vi "加速度_峰值.vi"(10 "信号X":dbl[](array[numeric]), 11 "n":i32) -> (3 "峰值":dbl)   [LabVIEW 2014]
uses:
  <vilib>/Analysis/NI_AAL_SigProc.lvlib
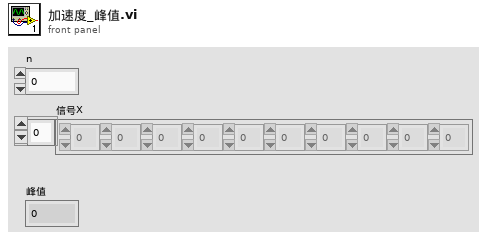
[diagram p1: front panel]
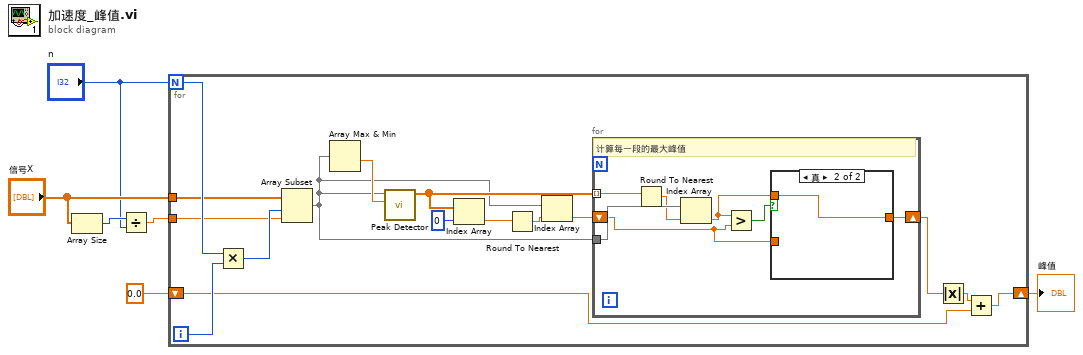
[diagram p0: block diagram]
diagram:
  n1 = Array Size(array="信号X") -> (size(s)=w3:i32)
  n2 = Divide(x=w3, y="n") -> (x/y=w1:dbl)
  n3 = for {
    N: "n" -> [w20]
    shift-right: [w12] -> w5
    shift-left: 0.0 -> [w11]
    tunnel: "信号X" -> [w8]
    tunnel: w1 -> [w7]
    i -> [w22]
    n4 = Multiply(x=w20, y=w22) -> (x*y=w21:i32)
    n5 = Array Subset(array=w8, index=w21, length=w7) -> (w16:dbl[])
    n6 = Array Max & Min(array=w16) -> (min value=w19:dbl)  [unwired: 3 out]
    n7 = call <vilib>:"Peak Detector.vi"("threshold"=w19, "X"=w16) -> ("Locations"=w18:dbl[])  [unwired: 5 in, 4 out]
    n8 = Index Array(array=w18, index=0 ("索引")) -> (element=w15:dbl)
    n9 = Round To Nearest(number=w15) -> (nearest integer value=w14:dbl)
    n10 = Index Array(array=w16, index=w14) -> (element=w13:dbl)
    n11 = for {
      tunnel: w18 -> [w29] mode=indexing
      tunnel: w16 -> [w28]
      shift-right: [w24] -> w10
      shift-left: w13 -> [w23]
      # "计算每一段的最大峰值"
      n12 = Round To Nearest(number=w29) -> (nearest integer value=w27:dbl)
      n13 = Index Array(array=w28, index=w27) -> (element=w25:dbl)
      n14 = Greater?(x=w25, y=w23) -> (0:w26:bool)
      n15 = case shown="真" w26 {
        tunnel: w25 -> [_ w31]
        tunnel: [w30 w31] -> w24
        tunnel: w23 -> [w30 _]
        frame False {
        }
        frame True {
        }
      }
    }
    n16 = Absolute Value(x=w10) -> (abs(x)=w9:dbl)
    n17 = Add(x=w9, y=w11) -> (x+y=w12:dbl)
  }
  "峰值" <- w5
